vi "MKS670_1000_alarm.vi"(3 "enabled":bool=TRUE, 5 "HIHI":dbl=700.0 format="%.1f", 7 "HI":dbl=500.0 format="%.1f", 8 "time_last_alarm_in":timestamp, 10 "readout_status":bool=TRUE, 11 "P":dbl) -> (0 "time_last_alarm_out":timestamp, 2 "alarm_status":u32(colorbox))   [LabVIEW 2019]
panel:
  out "message":string
  in  "interval":dbl=600.0
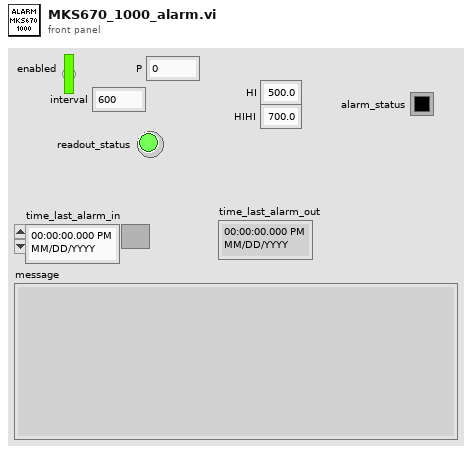
[diagram p1: front panel]
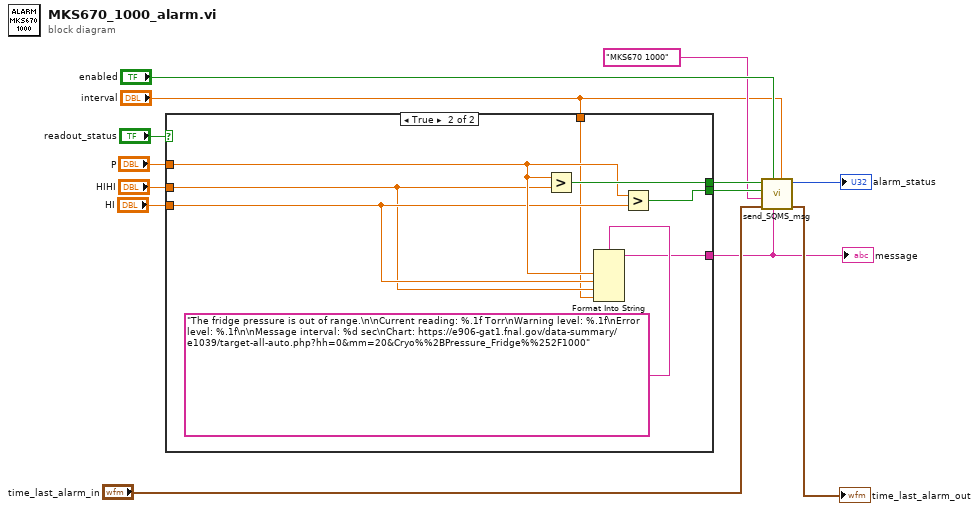
[diagram p0: block diagram]
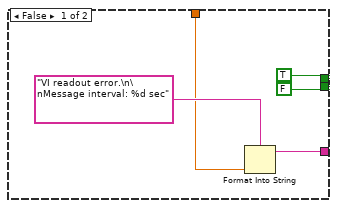
[diagram p2: hidden frame]
diagram:
  n1 = case shown="True" "readout_status" {
    tunnel: [TRUE w25] -> w12
    tunnel: [FALSE w24] -> w11
    tunnel: "HI" -> [_ w22]
    tunnel: "HIHI" -> [_ w21]
    tunnel: [w15 w19] -> w5
    tunnel: "P" -> [_ w23]
    tunnel: "interval" -> [w14 w20]
    frame False {
      n2 = Format Into String(format string="VI readout error.\n\nMessage interval: %d sec" ("msg"), w14) -> (resulting string=w15:string)  [unwired: 2 in, 1 out]
    }
    frame True {
      n3 = Greater?(x=w23, y=w21) -> (0:w25:bool)
      n4 = Format Into String(format string="The fridge pressure is out of range.\n\nCurrent reading: %.1f Torr\nWarning level: %.1f\nError       level: %.1f\n\nMessage interval: %d sec\nChart: https://e906-gat1.fnal.gov/data-summary/e1039/target-all-auto.php?hh=0&mm=20&Cryo%%2BPressure_Fridge%%252F1000" ("msg"), w23, w22, w21, w20) -> (resulting string=w19:string)  [unwired: 2 in, 1 out]
      n5 = Greater?(x=w23, y=w22) -> (0:w24:bool)
    }
  }
  "message" <- w5
  n6 = call "send_SQMS_msg.vi"("alarm_interval"="interval", "msg"=w5, "enabled"="enabled", "time_last_alarm_in"="time_last_alarm_in", "title"="MKS670 1000", "warning"=w11, "error"=w12) -> ("time_last_alarm_out"=→"time_last_alarm_out":timestamp, "alarm_status"=→"alarm_status":u32)  [unwired: 2 in, 1 out]
